vi "AsyncEngine.CANProtectionAndCounter.vi"(10 "Parameters":variant, 11 "Process":refnum<class "Process.lvclass">) -> ()   [LabVIEW 2015, in "Protection and Counter Addon Engine.lvlib"]
uses:
  Protection and Counter Addon Engine.lvlib
  <vilib>/NI/NIVS Inline Async API/_VS Inline Async API/Process/Process.lvclass
  Types/RT Async Engine Variables.ctl
  SubModules/Frame Protection Support/Source/Engine/Types/RT Frame Settings.ctl
  SubModules/Frame Protection Support/Source/Shared/Types/Exported Frame Type.ctl
  SubModules/Frame Protection Support/Source/Engine/Types/RT Protection Configuration.ctl
  SubModules/Frame Protection Support/Source/Shared/Types/Protection Type.ctl
  SubModules/Frame Protection Support/Source/Shared/Types/XNET Signal Configuration.ctl
  SubModules/Frame Protection Support/Source/Shared/Types/Exported Counter Settings.ctl
  SubModules/Frame Protection Support/Source/Shared/Types/Exported Event Trigger Type.ctl
  SubModules/Frame Protection Support/Source/Shared/Types/Exported Frame Settings.ctl
  SubModules/Frame Protection Support/Source/Shared/Types/Exported Protection Settings.ctl
  SubModules/Frame Protection Support/Source/Shared/Types/Incoming Signal Info.ctl
  SubModules/Frame Protection Support/Source/Shared/Types/Exported Signal Settings.ctl
  Types/RT Data References.ctl
  <vilib>/NI/NIVS Inline Async API/_Data Access Engine/Data Access Engine/Types/Write.DVR.ctl
  <vilib>/NI/NIVS Inline Async API/_Data Access Engine/Access Type Classes/Write/Write.lvclass
  <vilib>/NI/NIVS Inline Async API/_Data Access Engine/Data Access Engine/Types/Read.DVR.ctl
  <vilib>/NI/NIVS Inline Async API/_Data Access Engine/Access Type Classes/Read/Read.lvclass
  Users/Public/Documents/National Instruments/NI VeriStand 2015/Projects/Delete_Test_PaC_Incoming/LabVIEW/Incoming Frame Info.ctl
  <vilib>/NI/NIVS Inline Async API/_VS Inline Async API/Process/Process.lvclass/Process.ctl
  <vilib>/Platform/TimedLoop/XDataNode/timing_clust.ctl
  <vilib>/Platform/TimedLoop/XDataNode/nitl_modes.ctl
  <vilib>/Platform/TimedLoop/XDataNode/wakeup.ctl
  <vilib>/NI/NIVS Inline Async API/_Data Access Engine/Access Type Classes/Read/Read.lvclass/Read.ctl
  <vilib>/NI/NIVS Inline Async API/_Data Access Engine/Access Type Classes/Write/Write.lvclass/Write.ctl
  <vilib>/NI/NIVS Inline Async API/_VS Inline Async API/Process/Data Member Access/Read Data Access.vi
  <vilib>/NI/NIVS Inline Async API/_VS Inline Async API/Error Handling Process/SubVIs/Error.ConvertArray.vi
  <vilib>/NI/NIVS Inline Async API/_Data Access Engine/Data Access Engine/Methods/Data.Processes.Execute.vi
  <vilib>/NI/NIVS Inline Async API/_Data Access Engine/Data Access Engine/Methods/Write.Data.vi
  SubModules/Frame Protection Support/Source/Engine/SubVIs/Calculate Counter And Protections Main.vi
  <vilib>/NI/NIVS Inline Async API/_Data Access Engine/Access Type Classes/Write/Write.ProcessData.vi
  <vilib>/NI/NIVS Inline Async API/_Data Access Engine/Data Access Engine/Methods/Read.Data.Detect.vi
  <vilib>/NI/NIVS Inline Async API/_Data Access Engine/Data Access Engine/Methods/Write.Data.Buffer.vi
  SubModules/Frame Protection Support/Source/Engine/SubVIs/Determine Transmission.vi
  SubModules/Frame Protection Support/Source/Engine/SubVIs/Determine Periodic.vi
  <vilib>/NI/NIVS Inline Async API/_Data Access Engine/Data Access Engine/Methods/Write.Data.Commit.vi
  <vilib>/NI/NIVS Inline Async API/_Data Access Engine/Access Type Classes/Read/Read.ProcessData.Detect.vi
  <vilib>/NI/NIVS Inline Async API/_Data Access Engine/Access Type Classes/Write/Write.Buffer.vi
  <vilib>/NI/NIVS Inline Async API/_Data Access Engine/Access Type Classes/Write/Write.Commit.vi
  <vilib>/xnet/xnet.llb/XNET Write.vi
  <vilib>/xnet/xnet.llb/XNET Write (Frame CAN).vi
  <vilib>/xnet/xnet.llb/XNET Convert.vi
  <vilib>/xnet/xnet.llb/XNET Convert (Signal to Frame CAN).vi
  <vilib>/xnet/xnet.llb/XNET Convert (Signal to Frame Raw).vi
  <vilib>/NI/NIVS Inline Async API/_Data Access Engine/Data Access Engine/Methods/Write.Lookup.vi
  <vilib>/NI/NIVS Inline Async API/_Data Access Engine/Data Access Engine/Methods/Read.Lookup.vi
  Shared/SubVIs/GUID Lookup.vi
  <vilib>/Platform/TimedLoop/XDataNode/XDataNode.xnode
  <vilib>/NI/NIVS Inline Async API/_Data Access Engine/Data Access Engine/Data Access Engine.lvclass
  SubModules/Frame Protection Support/Source/Shared/Protection and Counter Support Shared.lvlib
  SubModules/Frame Protection Support/Source/Engine/Protection and Counter Support Engine.lvlib
  Shared/Protection and Counter Addon Shared.lvlib
  <vilib>/NI VeriStand/Custom Device Tools/Custom Device Utility Library/Custom Device Utility Library.lvlib
  <vilib>/Platform/TimedLoop/XDataNode/XDNodeRunTimeDep.lvlib
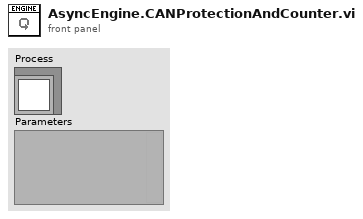
[diagram p1: front panel]
types:
  T1 = typedef "Protection and Counter Addon Engine.lvlib/Incoming Frame Info.ctl" = cluster{"data":cluster{"timestamp":timestamp[], "value":dbl[]}[], "Prev Frame Signal Values":dbl[], "Prev Frame Receive Time":timestamp, "Delta t":dbl}
  T2 = typedef "Protection and Counter Addon Engine.lvlib/RT Data References.ctl" = cluster{"ProtectionsAndCounters.Ref":T3, "Signals.Ref":T4, "Status.Ref":T3}
  T3 = typedef "Data Access Engine.lvlib/Data Access Engine.lvclass/Write.DVR.ctl" = refnum<data-value>
  T4 = typedef "Data Access Engine.lvlib/Data Access Engine.lvclass/Read.DVR.ctl" = refnum<data-value>
  T5 = typedef "Protection and Counter Addon Engine.lvlib/RT Async Engine Variables.ctl" = cluster{"Priority":i32, "CAN Session":refnum<k21>, "Frame Count":i32, "Frames":T6[], "FPGA Session":u32, "Incoming Frame Session":refnum<k21>, "Incoming Session Invalid":bool, "Incoming Frames":T13[], "Signal Values":dbl[], "Incoming Signal Info":T15}
  T6 = typedef "Protection and Counter Support Engine.lvlib/RT Frame Settings.ctl" = cluster{"Type":T7, "Frame ID":u32, "Payload Length":u32, "VS Offset":i32, "VS Length":i32, "Frame Conversion":refnum<k21>, "Frame.PrevData":dbl[], "Generation Period":u32, "Time Since Last Generation":u32, "Generation Iterations":u32, "Generation Counter":u32, "Has Protection?":bool, "Protection Configurations":T8[], "Has Counter?":bool, "Counter Configurations":T11[], "Has Disable?":bool, "Disable VS Index":i32, "Transmit Trigger":T12, "Trigger VS Index":i32}
  T7 = typedef "Protection and Counter Support Shared.lvlib/Exported Frame Type.ctl" = enum16{"Periodic", "Event", "Periodic/Event"}
  T8 = typedef "Protection and Counter Support Engine.lvlib/RT Protection Configuration.ctl" = cluster{"Protection Frame Index":i32, "Protection Type":T9, "Data Indeces":i32[], "Initialized Data Array":dbl[], "Check Sum Conversion":refnum<k21>, "CRC Channels":T10[], "Protection VS Index":i32}
  T9 = typedef "Protection and Counter Support Shared.lvlib/Protection Type.ctl" = enum16{"Arb ID + Bytes Checksum with Inversion", "Arb ID + Bytes CRC with Inversion", "Reversed Raw Signal Checksum with Inversion"}
  T10 = typedef "Protection and Counter Support Shared.lvlib/XNET Signal Configuration.ctl" = cluster{"Start Bit":i32, "Name":string, "Number of bits":i32, "Scale":dbl, "Offset":dbl, "Data Type":u32}
  T11 = typedef "Protection and Counter Support Shared.lvlib/Exported Counter Settings.ctl" = cluster{"Counter Frame Index":i32, "Max Count":dbl, "Counter VS Index":i32}
  T12 = typedef "Protection and Counter Support Shared.lvlib/Exported Event Trigger Type.ctl" = enum16{"Channel value change", "Trigger channel (not zero)", "Channel value change or trigger channel (not zero)", "Trigger channel (any value change)", "Channel value change or trigger channel (any value change)"}
  T13 = typedef "Protection and Counter Support Shared.lvlib/Exported Frame Settings.ctl" = cluster{"Type":T7, "Frame ID":u32, "Payload Length":u32, "Signal XNET Paths":string[], "Frame.PrevData":dbl[], "VS Offset":i32, "VS Length":i32, "Generation Period":u32, "Has Protection?":bool, "Protection Configurations":T14[], "Has Counter":bool, "Counter Configurations":T11[], "Has Disable?":bool, "Disable VS Index":i32, "Transmit Trigger":T12, "Trigger VS Index":i32}
  T14 = typedef "Protection and Counter Support Shared.lvlib/Exported Protection Settings.ctl" = cluster{"Protection Frame Index":i32, "Protection Type":T9, "Data Indeces":i32[], "Initialized Data Array":dbl[], "Protection Signal XNET Paths":string[], "CRC Channels":T10[], "Protection VS Update Index":i32}
  T15 = typedef "Protection and Counter Support Shared.lvlib/Incoming Signal Info.ctl" = cluster{"Signal Settings Out":T16[], "Signal.PrevData":dbl[], "Signal Names":string[]}
  T16 = typedef "Protection and Counter Support Shared.lvlib/Exported Signal Settings.ctl" = cluster{"Is Protection":bool, "Is Counter":bool, "Signal Name":string, "Counter Configuration":T11, "Protection Configuration":T14, "Valid_Sig_Ref_Index":i32}
  T17 = typedef "XDNodeRunTimeDep.lvlib/timing_clust.ctl" = cluster{"Expected End [f-1]":u64, "Actual End [f-1]":u64, "Finished Late? [f-1]":bool, "Expected End [i-1]":u64, "Actual End [i-1]":u64, "Finished Late? [i-1]":bool, "Expected Start [i]":u64, "Actual Start [i]":u64, "Expected Start [f]":u64, "Actual Start [f]":u64, "Source Name":string, "Structure Name":string, "Period":i64, "Deadline":i64, "Offset":i64, "Start":i64, "Priority":i32, "Timeout":i32, "Mode":T18, "Wakeup Reason":T19, "Error":errorcluster, "Source Type":string, "Secondary Source Type":string, "Global End Time":u64, "Global Start Time":u64, "Frame Duration":u64, "Iteration Duration":u64, "Assigned CPU":i32, "I/O Scan Engine Mode":u32}
  T18 = typedef "XDNodeRunTimeDep.lvlib/nitl_modes.ctl" = enum32{"No Change", "Process missed periods, maintain original phase", "Discard missed periods, maintain original phase", "Process missed periods, ignore original phase", "Discard missed periods, ignore original phase"}
  T19 = typedef "XDNodeRunTimeDep.lvlib/wakeup.ctl" = enum32{"Normal", "Aborted", "Asynchronous wakeup", "Timing source error", "Timed loop error", "Timeout"}
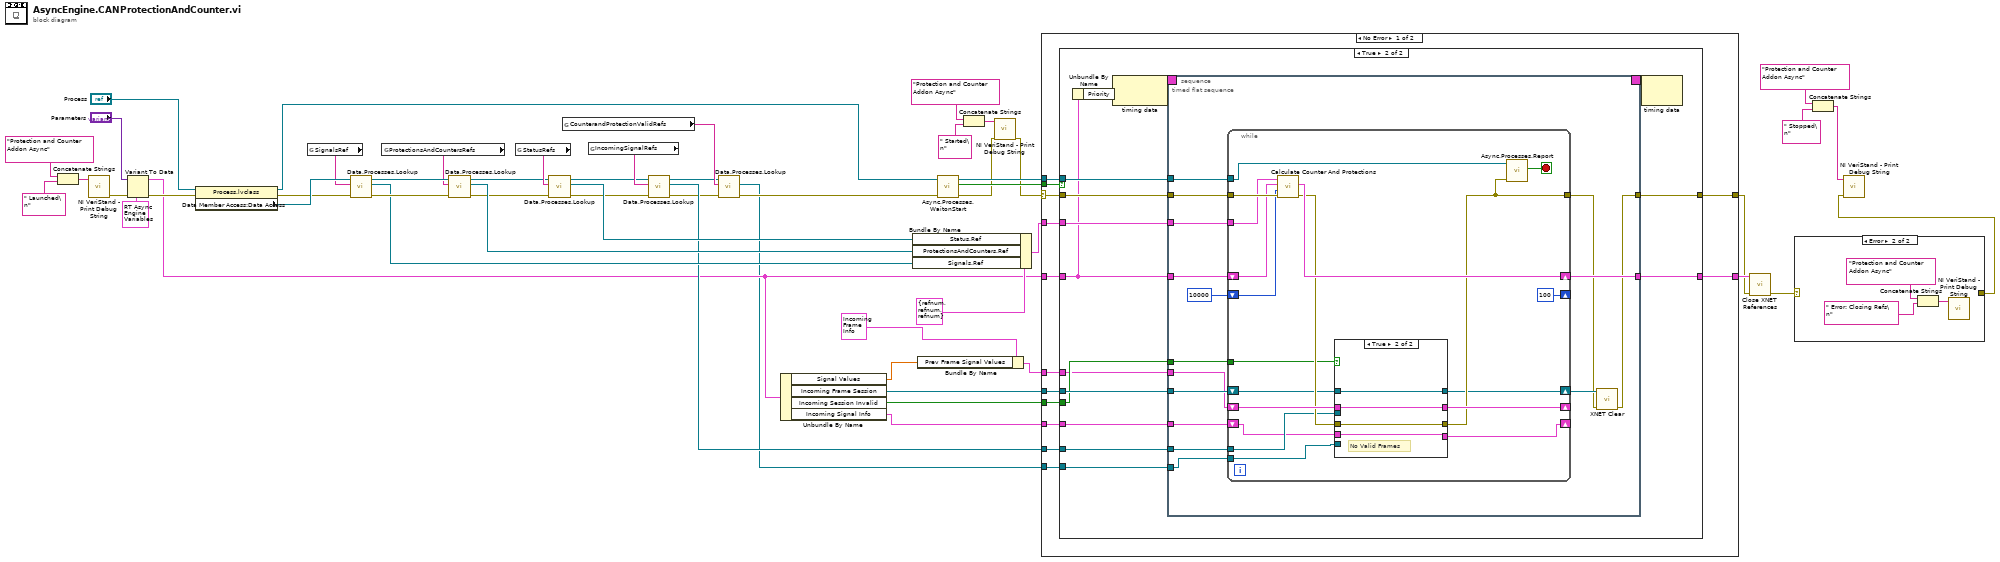
[diagram p0: block diagram]
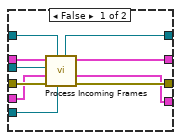
[diagram p4: hidden frame]
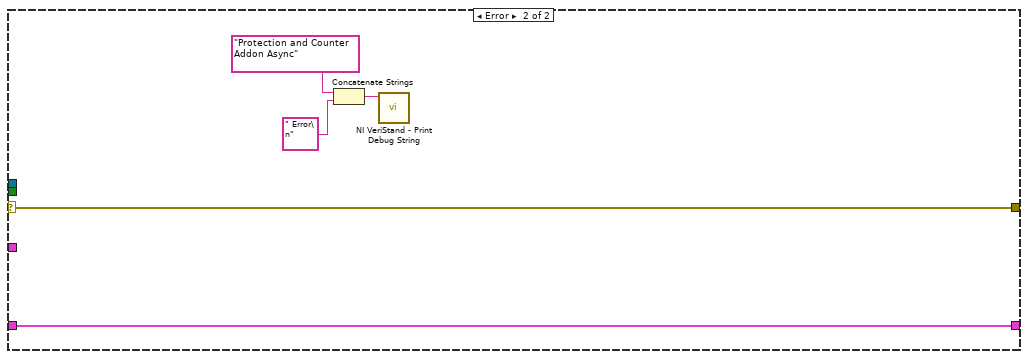
[diagram p5: hidden frame]
diagram:
  n1 = Concatenate Strings("Protection and Counter Addon Async" ("Debug String"), " Launched\n" ("string")) -> (w48:string)
  n2 = call <vilib>:"NI VeriStand - Print Debug String.vi"("Message"=w48) -> ("error out"=w46:errorcluster)  [unwired: 10 in]
  n3 = Variant To Data(error in=w46, type=T5 {"Priority"=100, "CAN Session"="", "Frame Count"=0, "Frames"=[], "FPGA Session"=0, "Incoming Frame Session"="", "Incoming Session Invalid"=FALSE, "Incoming Frames"=[], "Signal Values"=[], "Incoming Signal Info"={"Signal Settings Out"=[], "Signal.PrevData"=[], "Signal Names"=[]}} ("RT Configuration"), Variant="Parameters") -> (data=w12:T5, error out=w51:errorcluster)
  n4 = property class="Process.lvclass"(reference="Process", error in=w51) -> (reference out=w39:refnum<class "Process.lvclass">, error out=w43:errorcluster, "Data Member Access:Data Access"=w45:refnum<class "Data Access Engine.lvclass">)
  n5 = global read "GUID Lookup.vi" "SignalsRef"() -> (w41:string)
  n6 = call-poly <vilib>:"Data.Processes.Lookup.vi"("error in (no error)"=w43, "Name"=w41, "Data Access API in"=w45) -> ("error out"=w42:errorcluster, "Ref"=w37:T4, "Data Access API out"=w44:refnum<class "Data Access Engine.lvclass">)  [unwired: 5 in, 1 out]
  n7 = global read "GUID Lookup.vi" "ProtectionsAndCountersRefs"() -> (w40:string)
  n8 = call-poly <vilib>:"Data.Processes.Lookup.vi"("error in (no error)"=w42, "Name"=w40, "Data Access API in"=w44) -> ("error out"=w30:errorcluster, "Ref"=w36:T3, "Data Access API out"=w31:refnum<class "Data Access Engine.lvclass">)  [unwired: 5 in, 1 out]
  n9 = global read "GUID Lookup.vi" "StatusRefs"() -> (w32:string)
  n10 = call-poly <vilib>:"Data.Processes.Lookup.vi"("error in (no error)"=w30, "Name"=w32, "Data Access API in"=w31) -> ("error out"=w14:errorcluster, "Ref"=w29:T3, "Data Access API out"=w15:refnum<class "Data Access Engine.lvclass">)  [unwired: 5 in, 1 out]
  n11 = global read "GUID Lookup.vi" "CounterandProtectionValidRefs"() -> (w7:string)
  n12 = global read "GUID Lookup.vi" "IncomingSignalRefs"() -> (w16:string)
  n13 = call-poly <vilib>:"Data.Processes.Lookup.vi"("error in (no error)"=w14, "Name"=w16, "Data Access API in"=w15) -> ("error out"=w9:errorcluster, "Ref"=w13:T3, "Data Access API out"=w6:refnum<class "Data Access Engine.lvclass">)  [unwired: 5 in, 1 out]
  n14 = call-poly <vilib>:"Data.Processes.Lookup.vi"("error in (no error)"=w9, "Name"=w7, "Data Access API in"=w6) -> ("error out"=w8:errorcluster, "Ref"=w5:T3)  [unwired: 5 in, 2 out]
  n15 = Unbundle By Name(w12) -> ("Signal Values"=w2:dbl[], "Incoming Frame Session"=w11:refnum<k21>, "Incoming Session Invalid"=w10:bool, "Incoming Signal Info"=w1:T15)
  n16 = Bundle By Name(cluster=T2 {"ProtectionsAndCounters.Ref"=refnum, "Signals.Ref"=refnum, "Status.Ref"=refnum}, "Status.Ref"=w29, "ProtectionsAndCounters.Ref"=w36, "Signals.Ref"=w37) -> (w33:T2)
  n17 = Bundle By Name(cluster=T1 {"data"=[{"timestamp"=[], "value"=[]}, {"timestamp"=[], "value"=[]}, {"timestamp"=[], "value"=[]}, {"timestamp"=[], "value"=[]}], "Prev Frame Signal Values"=[], "Prev Frame Receive Time"=timestamp(0 s since 1904-01-01), "Delta t"=0.0} ("Incoming Frame Info Out"), "Prev Frame Signal Values"=w2) -> (w3:T1)
  n18 = call <vilib>:"Async.Processes.WaitonStart.vi"("error in (no error)"=w8, "Process"=w39) -> ("error out"=w25:errorcluster, "Execute"=w34:bool, "Process out"=w38:refnum<class "Process.lvclass">)  [unwired: 7 in]
  n19 = Concatenate Strings("Protection and Counter Addon Async" ("Debug String"), " Started\n" ("string")) -> (w27:string)
  n20 = call <vilib>:"NI VeriStand - Print Debug String.vi"("error in (no error)"=w25, "Message"=w27) -> ("error out"=w24:errorcluster)  [unwired: 9 in]
  n21 = case shown="No Error" w24 {
    selector: w24 -> [w62 w154]
    tunnel: w38 -> [w66 _]
    tunnel: w34 -> [w65 _]
    tunnel: w12 -> [w64 w150]
    tunnel: w33 -> [w63 _]
    tunnel: [w61 w154] -> w18
    tunnel: [w60 w150] -> w20
    tunnel: w13 -> [w59 _]
    tunnel: w11 -> [w58 _]
    tunnel: w10 -> [w57 _]
    tunnel: w5 -> [w56 _]
    tunnel: w3 -> [w55 _]
    tunnel: w1 -> [w54 _]
    frame No Error {
      n22 = case shown="True" w65 {
        tunnel: w66 -> [_ w83]
        tunnel: w64 -> [w67 w78]
        tunnel: w63 -> [_ w82]
        tunnel: w62 -> [w68 w81]
        tunnel: [w68 w80] -> w61
        tunnel: [w67 w79] -> w60
        tunnel: w59 -> [_ w74]
        tunnel: w58 -> [_ w73]
        tunnel: w57 -> [_ w72]
        tunnel: w56 -> [_ w71]
        tunnel: w55 -> [_ w70]
        tunnel: w54 -> [_ w69]
        frame False {
        }
        frame True {
          n23 = Unbundle By Name(w78) -> ("Priority"=w75:i32)
          n24 = node-c288(w75) -> (w77:T17)
          n25 = timed-sequence {
            timing: w77 -> [_]
            timing-out: [_] -> w76
            tunnel: w83 -> [w90]
            tunnel: w78 -> [w93]
            tunnel: w82 -> [w92]
            tunnel: w81 -> [w91]
            tunnel: [w95] -> w80
            tunnel: [w94] -> w79
            tunnel: w74 -> [w89]
            tunnel: w73 -> [w88]
            tunnel: w72 -> [w87]
            tunnel: w71 -> [w86]
            tunnel: w70 -> [w85]
            tunnel: w69 -> [w84]
            n26 = timed-flat-sequence {
              tunnel: [w100] -> w95
              tunnel: [w106] -> w94
              tunnel: w93 -> [w109]
              tunnel: w92 -> [w105]
              tunnel: w91 -> [w108]
              tunnel: w90 -> [w107]
              tunnel: w89 -> [w104]
              tunnel: w88 -> [w103]
              tunnel: w87 -> [w99]
              tunnel: w86 -> [w98]
              tunnel: w85 -> [w97]
              tunnel: w84 -> [w96]
              n27 = while {
                tunnel: w107 -> [w129]
                tunnel: w105 -> [w124]
                tunnel: w108 -> [w128]
                shift-right: [w125] -> w106
                shift-left: w109 -> [w127]
                tunnel: [w118] -> w101
                shift-right: [100 ("timeout ms")] -> _
                shift-left: 10000 ("timeout ms") -> [w123]
                shift-right: [w121] -> _
                shift-left: w97 -> [w120]
                tunnel: w104 -> [w117]
                shift-right: [w115] -> w102
                shift-left: w103 -> [w116]
                tunnel: w99 -> [w114]
                tunnel: w98 -> [w113]
                shift-right: [w111] -> _
                shift-left: w96 -> [w112]
                stop <- w126 stop-if-true
                n28 = call "Calculate Counter And Protections.vi"("error in (no error)"=w128, "timeout ms"=w123, "Async Settings"=w127, "Data Refs"=w124) -> ("error out"=w119:errorcluster, "Async Settings"=w125:T5)  [unwired: 6 in]
                n29 = case shown="True" w114 {
                  tunnel: [w139 w142] -> w121
                  tunnel: w120 -> [w138 w142]
                  tunnel: w119 -> [w137 w141]
                  tunnel: [w136 w141] -> w118
                  tunnel: w117 -> [w135 _]
                  tunnel: w116 -> [w134 w143]
                  tunnel: [w133 w143] -> w115
                  tunnel: w113 -> [w132 _]
                  tunnel: w112 -> [w131 w140]
                  tunnel: [w130 w140] -> w111
                  frame False {
                    n30 = call "Process Incoming Frames.vi"("SignalValidRefs"=w132, "Incoming Session"=w134, "error in"=w137, "Incoming Signal Info In"=w131, "Incoming Signal Refs"=w135, "Incoming Frame Info In"=w138) -> ("error out"=w136:errorcluster, "Incoming Signal Info Out"=w130:T15, "Incoming Frame Info Out"=w139:T1, "session out"=w133:refnum<k21>)  [unwired: 1 in, 1 out]
                  }
                  frame True {
                    # "No Valid Frames"
                  }
                }
                n31 = call <vilib>:"Async.Processes.Report.vi"("Error"=w118, "Process in"=w129) -> ("Stop"=w126:bool)  [unwired: 8 in, 1 out]
              }
              n32 = call <vilib>:"XNET Clear.vi"("session in"=w102, "error in (no error)"=w101) -> ("error out"=w100:errorcluster)  [unwired: 13 in]
            }
          }
          n33 = node-c288(w76) -> ()  [unwired: 1 out]
        }
      }
    }
    frame Error {
      n34 = Concatenate Strings("Protection and Counter Addon Async" ("Debug String"), " Error\n" ("string")) -> (w152:string)
      n35 = call <vilib>:"NI VeriStand - Print Debug String.vi"("Message"=w152) -> ()  [unwired: 10 in, 1 out]
    }
  }
  n36 = call "Close XNET References.vi"("error in (no error)"=w18, "RT Configuration"=w20) -> ("error out"=w19:errorcluster)  [unwired: 9 in]
  n37 = case shown="Error" w19 {
    selector: w19 -> [w155 _]
    tunnel: [w155 _] -> w17
    frame No Error {
    }
    frame Error {
      n38 = Concatenate Strings("Protection and Counter Addon Async" ("Debug String"), " Error: Closing Refs\n" ("string")) -> (w157:string)
      n39 = call <vilib>:"NI VeriStand - Print Debug String.vi"("Message"=w157) -> ()  [unwired: 10 in, 1 out]
    }
  }
  n40 = Concatenate Strings("Protection and Counter Addon Async" ("Debug String"), " Stopped\n" ("string")) -> (w22:string)
  n41 = call <vilib>:"NI VeriStand - Print Debug String.vi"("error in (no error)"=w17, "Message"=w22) -> ()  [unwired: 9 in, 1 out]
